vi "_Read.vi"(8 "error in (no error)":errorcluster, 11 "Temperature Controller Scientific Instruments in":refnum<class "Temperature Controller Scientific Instruments.lvclass">) -> (0 "error out":errorcluster, 2 "X array":T1, 3 "Temperature Controller Scientific Instruments out":refnum<class "Temperature Controller Scientific Instruments.lvclass">)   [LabVIEW 2023, in "Temperature Controller Scientific Instruments.lvclass"]
doc: "(Protected, Dynamic, Pure Virtual/Abstract) Perform a measurement and return one or more channels of data. Outsiders should not call this method, but instead the public \"Read Data.vi\"."
uses:
  Temperature Controller Scientific Instruments.lvclass
  Utility Classes/Readable/X array.ctl
  Utility Classes/Readable/X.ctl
  Utility Classes/Readable/Readable.lvclass
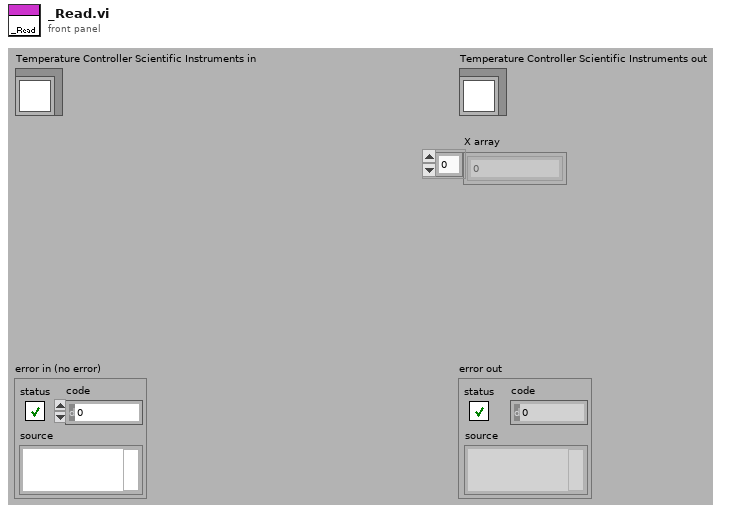
[diagram p1: front panel]
types:
  T1 = typedef "Readable.lvclass/X array.ctl" = T2[]
  T2 = typedef "Readable.lvclass/X.ctl" = dbl
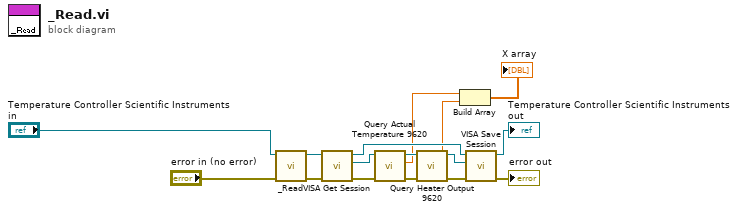
[diagram p0: block diagram]
diagram:
  n1 = call-parent "_Read.vi"("error in (no error)"="error in (no error)", "Readable in"="Temperature Controller Scientific Instruments in") -> ("error out"=w7:errorcluster, "Readable out"=w8:refnum<class "Temperature Controller Scientific Instruments.lvclass">)  [unwired: 7 in, 1 out]
  n2 = call-dynamic "VISA Get Session.vi"("error in (no error)"=w7, "Instrument.lvclass in"=w8) -> ("error out"=w11:errorcluster, "VISA Resource Name"=w14:refnum<visa-resource-name>, "Instrument.lvclass out"=w6:refnum<class "Temperature Controller Scientific Instruments.lvclass">)  [unwired: 7 out]
  n3 = call "Query Actual Temperature 9620.vi"("error in (no error)"=w11, "VISA resource name"=w14) -> ("error out"=w12:errorcluster, "Current actual temperature"=w3:dbl, "VISA resource name out"=w13:refnum<visa-resource-name>)  [unwired: 7 in]
  n4 = call "Query Heater Output 9620.vi"("error in (no error)"=w12, "VISA resource name"=w13) -> ("error out"=w10:errorcluster, "Current heater output"=w2:dbl, "VISA resource name out"=w9:refnum<visa-resource-name>)  [unwired: 7 in]
  n5 = Build Array(w3, w2) -> (→"X array":dbl[])
  n6 = call-dynamic "VISA Save Session.vi"("error in (no error)"=w10, "VISA Resource Name"=w9, "Instrument.lvclass in"=w6) -> ("error out"=→"error out":errorcluster, "Instrument.lvclass out"=→"Temperature Controller Scientific Instruments out":refnum<class "Temperature Controller Scientific Instruments.lvclass">)  [unwired: 7 out]
